vi "Increment request ID.vi"(11 "Message Loop Shift Register Data (in)":T1) -> (2 "New Request ID":u64, 3 "Message Loop Shift Register Data (out)":T1)   [LabVIEW 2020, in "wamplv.lvlib" / "WAMP Client.lvclass"]
uses:
  WAMP Client.lvclass
  TypeDef/Message Loop Shift Reg Data.ctl
  TypeDef/REGISTER Request Data.ctl
  API/TypeDefs/INVOCATION payload.ctl
  TypeDef/Success or error.ctl
  API/TypeDefs/Combined error.ctl
  API/TypeDefs/WAMP error.ctl
  TypeDef/Publish Requests Map.ctl
  TypeDef/PUBLISH Request Data.ctl
  TypeDef/PUBLISH result.ctl
  TypeDef/Endpoint Data.ctl
  TypeDef/CALL Request Map.ctl
  TypeDef/CALL Request Data.ctl
  API/TypeDefs/RESULT payload.ctl
  TypeDef/SUBSCRIBE Requests Map.ctl
  TypeDef/SUBSCRIBE Request Data.ctl
  TypeDef/Subscribe Result.ctl
  TypeDef/EVENT payload.ctl
  TypeDef/Subscriptions Map.ctl
  TypeDef/Subscription Details.ctl
  TypeDef/Unsubscribe Requests Map.ctl
  TypeDef/UNSUBSCRIBE Request Data.ctl
  TypeDef/UNSUBSCRIBE Result.ctl
  TypeDef/Unregister requests map.ctl
  TypeDef/Unregister request.ctl
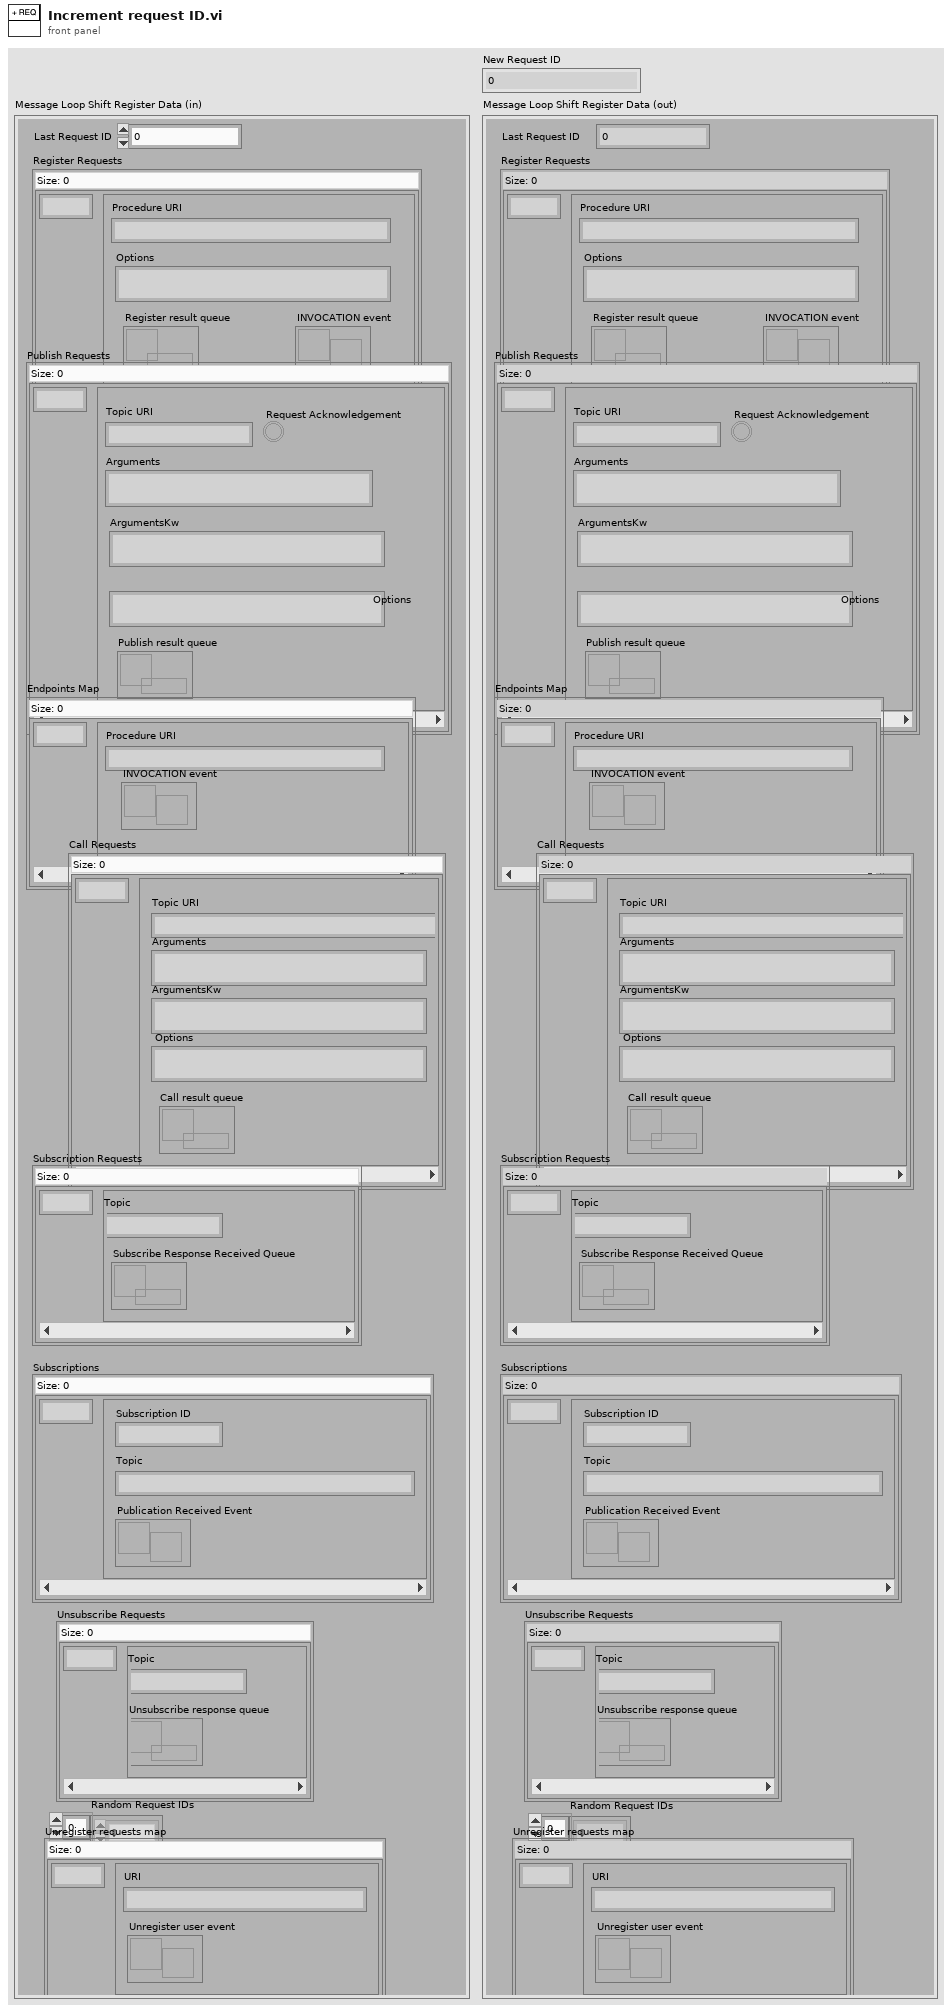
[diagram p1: front panel]
types:
  T1 = typedef "wamplv.lvlib/WAMP Client.lvclass/Message Loop Shift Reg Data.ctl" = cluster{"Last Request ID":u64, "Register Requests":map{u64, T2}, "Publish Requests":T3, "Endpoints Map":map{u64, T5}, "Call Requests":T6, "Subscription Requests":T8, "Subscriptions":T10, "Unsubscribe Requests":T12, "Random Request IDs":u64[], "Unregister requests map":T14}
  T2 = typedef "wamplv.lvlib/WAMP Client.lvclass/REGISTER Request Data.ctl" = cluster{"Procedure URI":string, "Options":string, "INVOCATION event":refnum<user-event>, "Register result queue":refnum<queue>}
  T3 = typedef "wamplv.lvlib/WAMP Client.lvclass/Publish Requests Map.ctl" = map{u64, T4}
  T4 = typedef "wamplv.lvlib/WAMP Client.lvclass/PUBLISH Request Data.ctl" = cluster{"Topic URI":string, "Arguments":string, "ArgumentsKw":string, "Request Acknowledgement":bool, "Options":string, "Publish result queue":refnum<queue>}
  T5 = typedef "wamplv.lvlib/WAMP Client.lvclass/Endpoint Data.ctl" = cluster{"Procedure URI":string, "INVOCATION event":refnum<user-event>}
  T6 = typedef "wamplv.lvlib/WAMP Client.lvclass/CALL Request Map.ctl" = map{u64, T7}
  T7 = typedef "wamplv.lvlib/WAMP Client.lvclass/CALL Request Data.ctl" = cluster{"Topic URI":string, "Arguments":string, "ArgumentsKw":string, "Options":string, "Call result queue":refnum<queue>}
  T8 = typedef "wamplv.lvlib/WAMP Client.lvclass/SUBSCRIBE Requests Map.ctl" = map{u64, T9}
  T9 = typedef "wamplv.lvlib/WAMP Client.lvclass/SUBSCRIBE Request Data.ctl" = cluster{"Topic":string, "Subscribe Response Received Queue":refnum<queue>}
  T10 = typedef "wamplv.lvlib/WAMP Client.lvclass/Subscriptions Map.ctl" = map{u64, T11}
  T11 = typedef "wamplv.lvlib/WAMP Client.lvclass/Subscription Details.ctl" = cluster{"Subscription ID":u64, "Topic":string, "Publication Received Event":refnum<user-event>}
  T12 = typedef "wamplv.lvlib/WAMP Client.lvclass/Unsubscribe Requests Map.ctl" = map{u64, T13}
  T13 = typedef "wamplv.lvlib/WAMP Client.lvclass/UNSUBSCRIBE Request Data.ctl" = cluster{"Topic":string, "Unsubscribe response queue":refnum<queue>}
  T14 = typedef "wamplv.lvlib/WAMP Client.lvclass/Unregister requests map.ctl" = map{u64, T15}
  T15 = typedef "wamplv.lvlib/WAMP Client.lvclass/Unregister request.ctl" = cluster{"URI":string, "Unregister user event":refnum<user-event>}
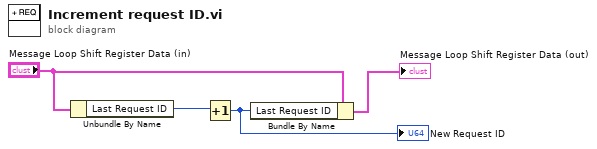
[diagram p0: block diagram]
diagram:
  n1 = Unbundle By Name("Message Loop Shift Register Data (in)") -> ("Last Request ID"=w2:u64)
  n2 = Increment(x=w2) -> (x+1=w1:u64)
  "New Request ID" <- w1
  n3 = Bundle By Name(cluster="Message Loop Shift Register Data (in)", "Last Request ID"=w1) -> (→"Message Loop Shift Register Data (out)":T1)
